vi "MKR1000 UDP Client.vi"() -> ()   [LabVIEW 2016]
uses:
  Typedef/Set channels.ctl
  Typedef/MKR1000 - States.ctl
  MKR1000.lvlib
panel:
  in  "Exit":bool
  out "Status":bool
  in  "Connect":bool
  in  "Server parameters":cluster{"IP":string, "Port":u16}={"IP"="192.168.1.5", "Port"=2390}
  in  "Local port":u16=3333
  in  "Set parameters":bool
  in  "Acquisition \nchannels":T1={"Chan 0"=TRUE, "Chan 1 1"=FALSE, "Chan 2"=FALSE, "Chan 3"=FALSE, "Chan 4 5"=FALSE, "Chan 5"=FALSE}
  in  "Acquisition \ninterval":i32=100 min=20 max=1000 step=10 format="%.0fms"
  in  "Acquire":bool
  out "Received Data":T2(graph)
  # "0. Modify the MKR1000 firmware to match with the SSID and the password of your network\n1. Set the IP of MKR1000 in the \"Server parameters\". Actually the firmware of the Genuino is made to overwrite the IP assigned by DHCP server with 192.168.1.5\n2. Press connect and wait for green led to turn on. If this doesn't happen you need to check that all devices are properly connected to the network\n3. Modify Acquisition channels and interval to match your needings and press \"Confirm parameters\".\n4. Press Acquire/Stop to start/stop the data transfer."
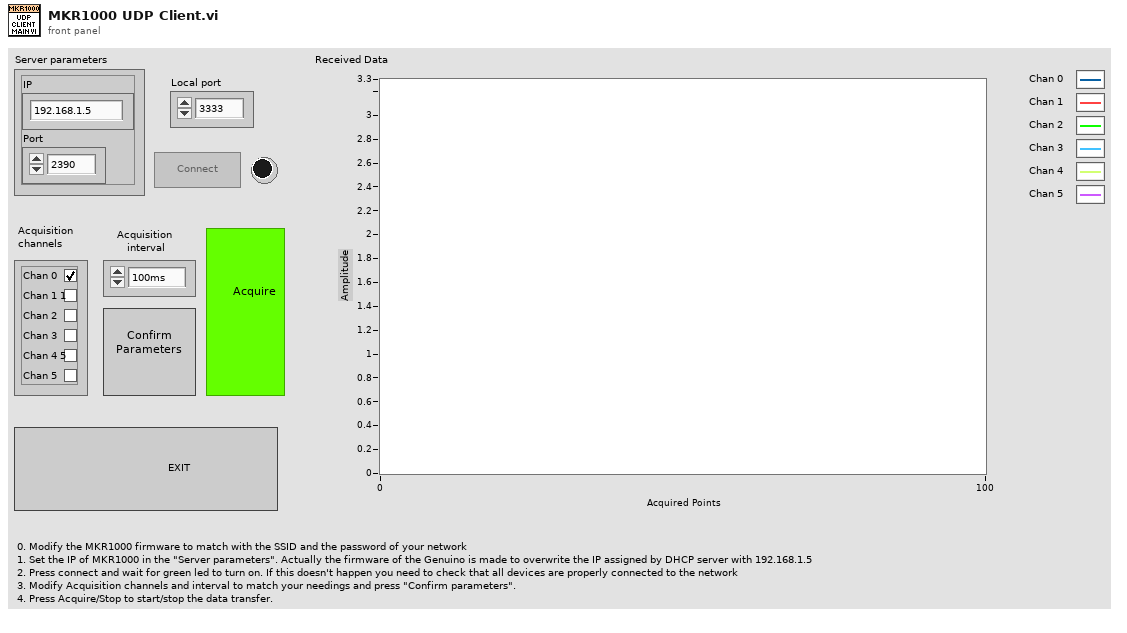
[diagram p1: front panel]
types:
  T1 = typedef "MKR1000.lvlib/Set channels.ctl" = cluster{"Chan 0":bool, "Chan 1 1":bool, "Chan 2":bool, "Chan 3":bool, "Chan 4 5":bool, "Chan 5":bool}
  T2 = cluster{"Numeric Control":sgl, "Numeric Control":sgl, "Numeric Control":sgl, "Numeric Control":sgl, "Numeric Control":sgl, "Numeric Control":sgl}
  T3 = typedef "MKR1000.lvlib/MKR1000 - States.ctl" = enum16{"Init", "Connect", "Idle", "Set parameters", "Acquire", "Get Data", "Stop"}
  T4 = enum8{"Enabled", "Disabled", "Disabled and Grayed Out"}
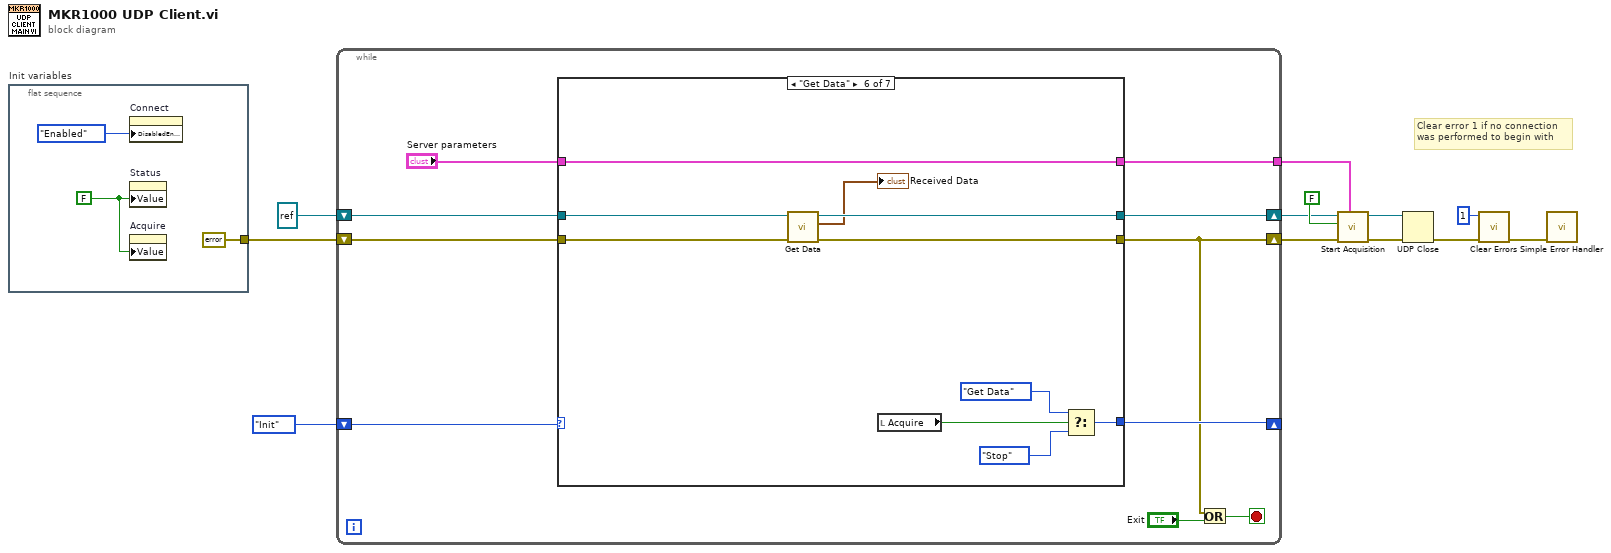
[diagram p0: block diagram]
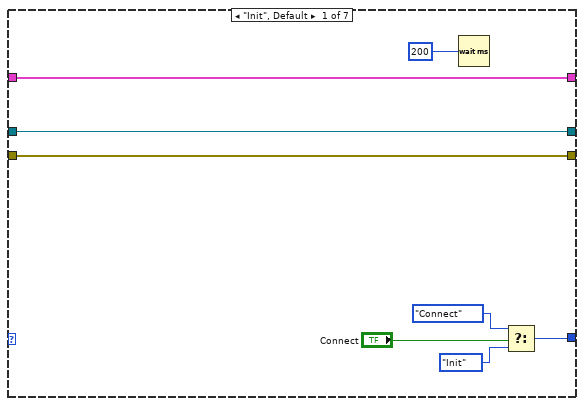
[diagram p2: hidden frame]
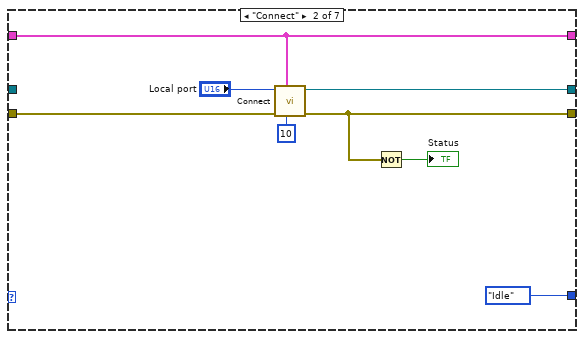
[diagram p3: hidden frame]
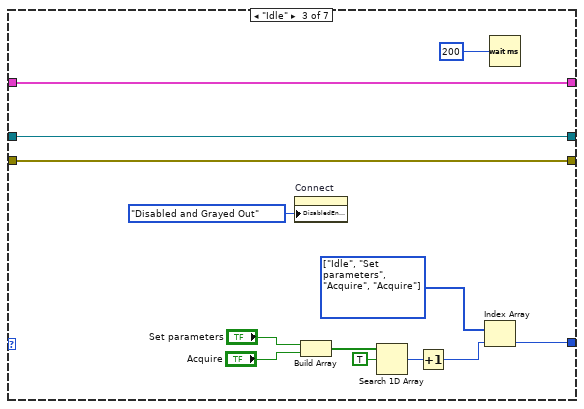
[diagram p4: hidden frame]
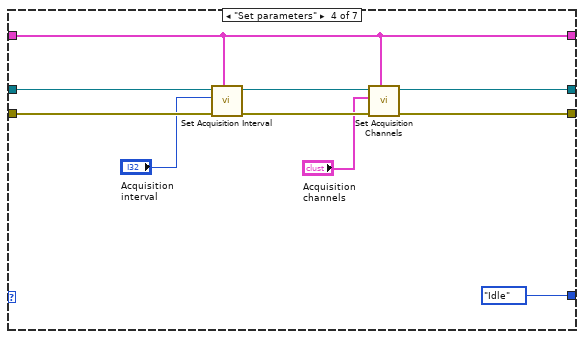
[diagram p5: hidden frame]
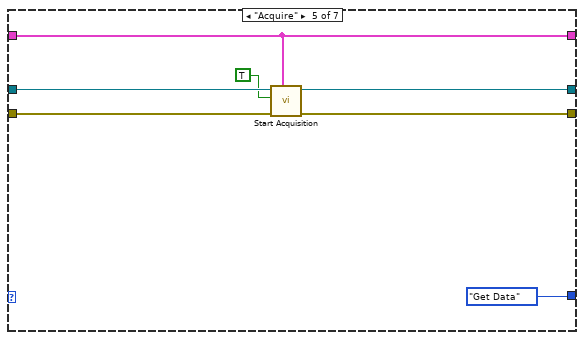
[diagram p6: hidden frame]
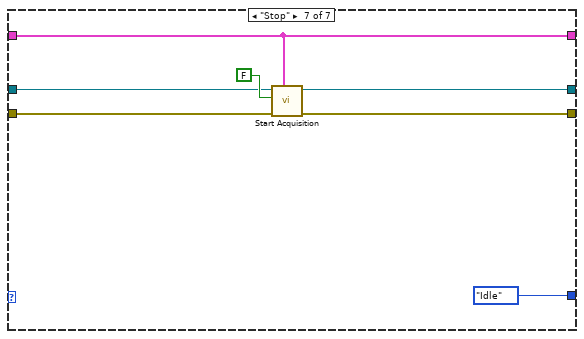
[diagram p7: hidden frame]
diagram:
  # "Clear error 1 if no connection\nwas performed to begin with"
  n1 = flat-sequence "Init variables" {
    tunnel: [errorcluster {"status"=FALSE, "code"=0, "source"=""} ("Error Out")] -> w10
    frame #0 {
      w14 = FALSE
      n2 = property on="Connect" class="Bool"("DisabledEnum"=T4."Enabled" ("Disabled")) -> ()  [unwired: 2 in, 2 out]
      n3 = property on="Status" class="Bool (strict)"("Value"=w14) -> ()  [unwired: 2 in, 2 out]
      n4 = property on="Acquire" class="Bool (strict)"("Value"=w14) -> ()  [unwired: 2 in, 2 out]
    }
  }
  n5 = while {
    shift-right: [w24] -> _
    shift-left: MKR1000_-_States."Init" -> [w25]
    shift-right: [w17] -> w3
    shift-left: w10 -> [w23]
    shift-right: [w22] -> w5
    shift-left: refnum<k16> refnum ("connection ID out") -> [w21]
    tunnel: [w16] -> w1
    stop <- w19 stop-if-true
    n6 = case shown="\"Get Data\"" w25 {
      tunnel: [w33 MKR1000_-_States."Idle" w46 MKR1000_-_States."Idle" MKR1000_-_States."Get Data" ("t") w76 MKR1000_-_States."Idle" ("f")] -> w24
      tunnel: [w30 w36 w54 w58 w68 w78 w85] -> w17
      tunnel: w23 -> [w30 w41 w54 w64 w70 w80 w84]
      tunnel: [w29 w40 w53 w60 w69 w79 w86] -> w22
      tunnel: w21 -> [w29 _ w53 w63 w71 w81 w87]
      tunnel: "Server parameters" -> [w26 w34 w42 w55 w65 w72 w82]
      tunnel: [w26 w34 w42 w55 w65 w72 w82] -> w16
      frame "Init", Default {
        n7 = Wait (ms)(milliseconds to wait=200) -> ()  [unwired: 1 out]
        n8 = Select(t=MKR1000_-_States."Connect", s="Connect", f=MKR1000_-_States."Init") -> (s? t:f=w33:T3)
      }
      frame "Connect" {
        n9 = call "Connect.vi"("N attempts"=10, "Server parameters"=w34, "Error In"=w41, "Local port"="Local port") -> ("Error Out"=w36:errorcluster, "connection ID out"=w40:refnum<k16>)  [unwired: 6 in]
        n10 = Not(x=w36) -> (.not. x?=→"Status":bool)
      }
      frame "Idle" {
        w47 = T3[] [enum."Idle", enum."Set parameters", enum."Acquire", enum."Acquire"] items=["Init", "Connect", "Idle", "Set parameters", "Acquire", "Get Data", "Stop"]
        n11 = property on="Connect" class="Bool"("DisabledEnum"=T4."Disabled and Grayed Out" ("Disabled")) -> ()  [unwired: 2 in, 2 out]
        n12 = Build Array("Set parameters", "Acquire") -> (w51:bool[])
        n13 = Search 1D Array(1D array=w51, element=TRUE) -> (index of element=w49:i32)  [unwired: 1 in]
        n14 = Increment(x=w49) -> (x+1=w48:i32)
        n15 = Index Array(array=w47, index=w48) -> (element=w46:T3)
        n16 = Wait (ms)(milliseconds to wait=200) -> ()  [unwired: 1 out]
      }
      frame "Set parameters" {
        n17 = call "Set Acquisition Interval.vi"("Client parameters"=w55, "Error In"=w64, "Acquisition interval [ms]"="Acquisition \ninterval", "connection ID"=w63) -> ("Error Out"=w59:errorcluster, "connection ID out"=w61:refnum<k16>)  [unwired: 6 in]
        n18 = call "Set Acquisition Channels.vi"("Client parameters"=w55, "Error In"=w59, "Acquisition channels"="Acquisition \nchannels", "connection ID"=w61) -> ("Error Out"=w58:errorcluster, "connection ID out"=w60:refnum<k16>)  [unwired: 6 in]
      }
      frame "Acquire" {
        n19 = call "Start Acquisition.vi"("Client parameters"=w65, "Error In"=w70, "Acquire"=TRUE, "connection ID"=w71) -> ("Error Out"=w68:errorcluster, "connection ID out"=w69:refnum<k16>)  [unwired: 6 in]
      }
      frame "Get Data" {
        n20 = call "Get Data.vi"("Error In"=w80, "connection ID"=w81) -> ("Error Out"=w78:errorcluster, "Data output"=→"Received Data":T2, "connection ID out"=w79:refnum<k16>)  [unwired: 7 in]
        n21 = local read "Acquire"() -> (w73:bool)
        n22 = Select(t=MKR1000_-_States."Get Data", s=w73, f=MKR1000_-_States."Stop") -> (s? t:f=w76:T3)
      }
      frame "Stop" {
        n23 = call "Start Acquisition.vi"("Client parameters"=w82, "Error In"=w84, "Acquire"=FALSE, "connection ID"=w87) -> ("Error Out"=w85:errorcluster, "connection ID out"=w86:refnum<k16>)  [unwired: 6 in]
      }
    }
    n24 = Or(x=w17, y="Exit") -> (x .or. y?=w19:bool)
  }
  n25 = call "Start Acquisition.vi"("Client parameters"=w1, "Error In"=w3, "Acquire"=FALSE, "connection ID"=w5) -> ("Error Out"=w2:errorcluster, "connection ID out"=w4:refnum<k16>)  [unwired: 6 in]
  n26 = UDP Close(connection ID=w4, 8:w2) -> (error out=w9:errorcluster)  [unwired: 1 out]
  n27 = call <vilib>:"Clear Errors.vi"("error in (no error)"=w9, "specific error code to clear (0: all)"=1) -> ("error out"=w8:errorcluster)  [unwired: 4 in, 1 out]
  n28 = call <vilib>:"Simple Error Handler.vi"("error in (no error)"=w8) -> ()  [unwired: 1 in, 8 out]
